vi "57XX.vi"(5 "Frequency (125 Hz) (0, 10 - 10e3)":dbl=125.0 format="%#_6p", 7 "Voltage/Current (V, V rms, A) (1)":dbl=1.0, 8 "error in (no error)":errorcluster, 9 "ext. Guard (F)":bool, 10 "Current (F)":bool, 11 "Phase Lock (T)":bool=TRUE) -> (0 "error out":errorcluster)   [LabVIEW 2019, in "ACSVcontrol-driver.lvlib"]
doc: "Set function generator. Init True will change the phase without a new initialisation, i.e. without switching to standby mode."
uses:
  ACSVcontrol-driver.lvlib
  Private/Type definitions/Command.ctl
  Private/Type definitions/Status.ctl
  Private/Globals.vi
  <vilib>/Utility/error.llb/Error Cluster From Error Code.vi
  <vilib>/ErrorRing/Error Ring.xnode
panel:
  in  "number format string":string="%.6f"
  out "resulting string":string
  # ".7 is too much,\nworking maximum is .6"
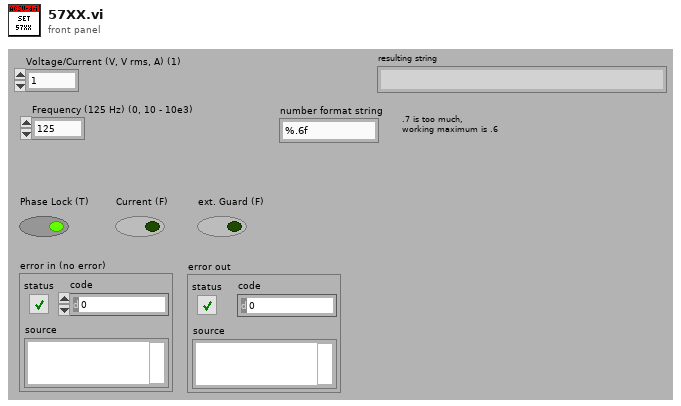
[diagram p1: front panel]
types:
  T1 = typedef "ACSVcontrol-driver.lvlib/Status.ctl" = enum16{"waiting", "processing", "error command", "Set_PJVS-Done", "Set_Mux-Done", "Set_Mux-Error", "Set_57XX-Done", "Set_57XX-Error", "Set_Gen-Done", "Set_Gen-Error", "Set_Synthesizer-Done", "Set_Synthesizer-Error", "Read_Nano-Done", "Read_Sampler-Done", "Read_Sampler-Error", "Read_Sensors-Done"}
  T2 = typedef "ACSVcontrol-driver.lvlib/Command.ctl" = enum16{"Set_PJVS", "Set_Mux", "Set_57XX", "Set_Gen", "Set_Synthesizer", "Read_Nulldetector", "Read_Sampler", "Read_Sensors"}
  T3 = typedef "ACSVcontrol-driver.lvlib/Timeouts.ctl" = cluster{"TCP Read & Write (ms)":i32, "Sensors readout":i32, "PJVS setup":i32, "Nullmeter readout":i32, "Multiplexer setup":i32, "57XX setup":i32, "Generator setup":i32, "Synthesizer setup":i32, "Sampler readout":i32}
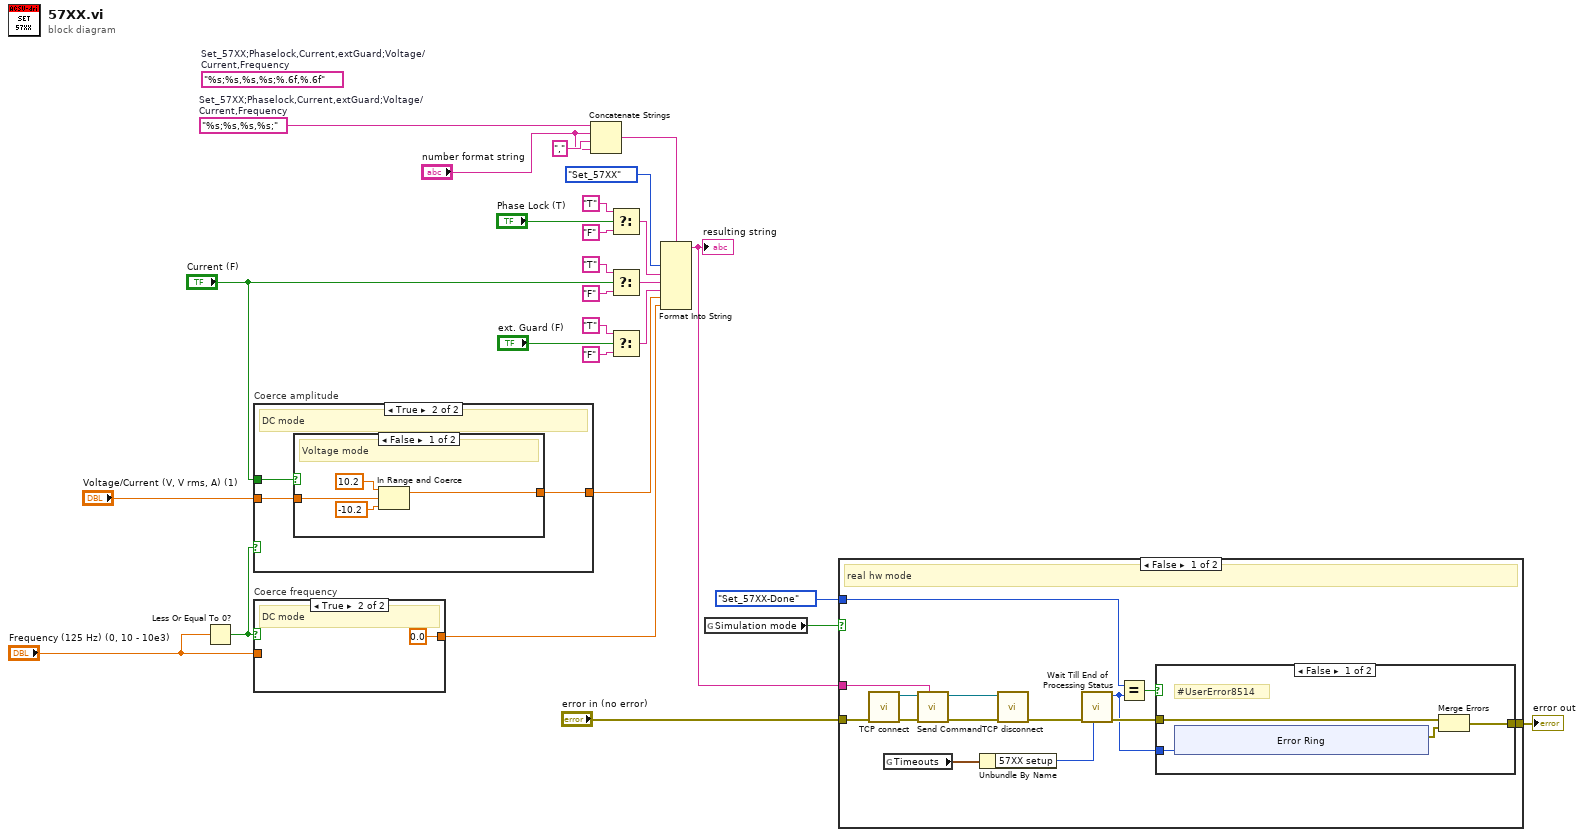
[diagram p0: block diagram]
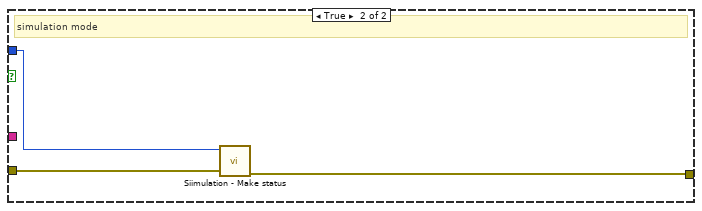
[diagram p3: hidden frame]
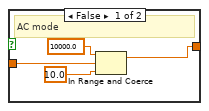
[diagram p4: hidden frame]
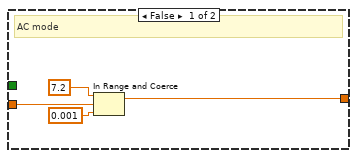
[diagram p5: hidden frame]
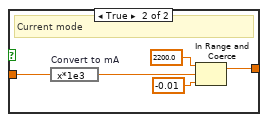
[diagram p6: hidden frame]
diagram:
  w6 = "%s;%s,%s,%s;"  # Set_57XX;Phaselock,Current,extGuard;Voltage/Current,Frequency
  (unwired) "%s;%s,%s,%s;%.6f,%.6f"  # Set_57XX;Phaselock,Current,extGuard;Voltage/Current,Frequency
  n1 = Less Or Equal To 0?(x="Frequency (125 Hz) (0, 10 - 10e3)") -> (x <= 0?=w3:bool)
  n2 = case "Coerce amplitude" shown="True" w3 {
    tunnel: "Voltage/Current (V, V rms, A) (1)" -> [w30 w34]
    tunnel: [w31 w33] -> w18
    tunnel: "Current (F)" -> [_ w32]
    frame False {
      # "AC mode"
      n3 = In Range and Coerce(upper limit=7.2 ("lower limit"), x=w30, lower limit=0.001) -> (coerced(x)=w31:dbl)  [unwired: 1 out]
    }
    frame True {
      # "DC mode"
      n4 = case shown="False" w32 {
        tunnel: w34 -> [w38 w40]
        tunnel: [w37 w41] -> w33
        frame False {
          # "Voltage mode"
          n5 = In Range and Coerce(upper limit=10.2 ("lower limit"), x=w38, lower limit=-10.2) -> (coerced(x)=w37:dbl)  [unwired: 1 out]
        }
        frame True {
          # "Current mode"
          n6 = expression code="x*1e3" "Convert to mA"(w40) -> (w39:dbl)
          n7 = In Range and Coerce(upper limit=2200.0, x=w39, lower limit=-0.01) -> (coerced(x)=w41:dbl)  [unwired: 1 out]
        }
      }
    }
  }
  n8 = case "Coerce frequency" shown="True" w3 {
    tunnel: [w45 0.0 ("upper limit")] -> w17
    tunnel: "Frequency (125 Hz) (0, 10 - 10e3)" -> [w44 _]
    frame False {
      # "AC mode"
      n9 = In Range and Coerce(upper limit=10000.0, x=w44, lower limit=10.0) -> (coerced(x)=w45:dbl)  [unwired: 1 out]
    }
    frame True {
      # "DC mode"
    }
  }
  n10 = Concatenate Strings(w6, "number format string", "," ("string"), "number format string") -> (w14:string)
  n11 = Select(t="T" ("format string"), s="Phase Lock (T)", f="F" ("format string")) -> (s? t:f=w22:string)
  n12 = Select(t="T" ("format string"), s="Current (F)", f="F" ("format string")) -> (s? t:f=w21:string)
  n13 = Select(t="T" ("format string"), s="ext. Guard (F)", f="F" ("format string")) -> (s? t:f=w7:string)
  n14 = Format Into String(format string=w14, Command."Set_57XX" ("Command"), w22, w21, w7, w18, w17) -> (resulting string=w12:string)  [unwired: 2 in, 1 out]
  "resulting string" <- w12
  n15 = global read "Globals.vi" "Simulation mode"() -> (w2:bool)
  n16 = case shown="False" w2 {
    tunnel: "error in (no error)" -> [w62 w77]
    tunnel: [w56 w76] -> w13
    tunnel: w12 -> [w51 _]
    tunnel: Status."Set_57XX-Done" ("x") -> [w49 w75]
    frame False {
      # "real hw mode"
      n17 = call "TCP connect.vi"("error in (no error)"=w62) -> ("error out"=w59:errorcluster, "connection ID"=w58:refnum<k5>)  [unwired: 9 in]
      n18 = global read "Globals.vi" "Timeouts"() -> (w50:T3)
      n19 = call "Send Command.vi"("Command"=w51, "error in (no error)"=w59, "connection ID"=w58) -> ("error out"=w60:errorcluster, "connection ID out"=w61:refnum<k5>)  [unwired: 7 in]
      n20 = Unbundle By Name(w50) -> ("57XX setup"=w52:i32)
      n21 = call "TCP disconnect.vi"("error in (no error)"=w60, "connection ID"=w61) -> ("error out"=w57:errorcluster)  [unwired: 9 in]
      n22 = call "Wait Till End of Processing Status.vi"("Loop Timeout (ms) (5000)"=w52, "error in (no error)"=w57) -> ("error out"=w55:errorcluster, "Last Status"=w53:T1)  [unwired: 8 in]
      n23 = Equal?(x=w49, y=w53) -> (x = y?=w54:bool)
      n24 = case shown="False" w54 {
        tunnel: w55 -> [w66 w74]
        tunnel: [w64 w74] -> w56
        tunnel: w53 -> [w63 _]
        frame False {
          # "#UserError8514"
          n25 = xnode "Error Ring"("parameter 0"=w63) -> ("error out"=w65:errorcluster)
          n26 = Merge Errors(w66, w65) -> (w64:errorcluster)
        }
        frame True {
        }
      }
    }
    frame True {
      # "simulation mode"
      n27 = call "Siimulation - Make status.vi"("error in (no error)"=w77, "Status"=w75) -> ("error out"=w76:errorcluster)  [unwired: 8 in, 1 out]
    }
  }
  "error out" <- w13
